vi "setup_id_from_ctlref.vi"(6 "error in":errorcluster, 7 "Ctl Refnum":refnum<vi>) -> (0 "error out":errorcluster, 1 "setup ID":u16)   [LabVIEW 2016]
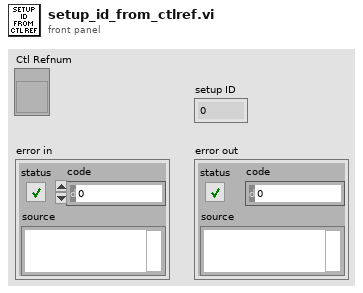
[diagram p1: front panel]
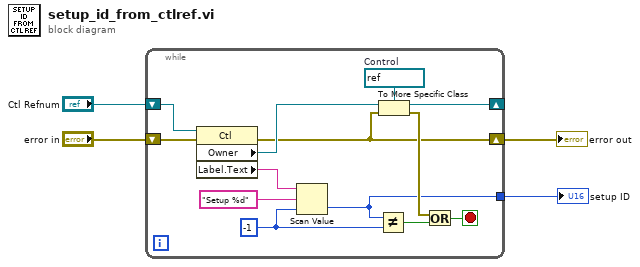
[diagram p0: block diagram]
diagram:
  n1 = while {
    shift-right: [w16] -> _
    shift-left: "Ctl Refnum" -> [w14]
    shift-right: [w8] -> w2
    shift-left: "error in" -> [w15]
    tunnel: [w5] -> w3
    stop <- w11 stop-if-true
    w6 = -1 ("default (0 dbl)")
    w17 = refnum<vi> refnum  # Control
    n2 = property class="Ctl"(reference=w14, error in=w15) -> (error out=w8:errorcluster, "Owner"=w10:refnum<vi>, "Label.Text"=w7:string)  [unwired: 1 out]
    n3 = Scan Value(string=w7, format string="Setup %d", default (0 dbl)=w6) -> (value=w5:i32)  [unwired: 1 out]
    n4 = Not Equal?(x=w5, y=w6) -> (x != y?=w13:bool)
    n5 = To More Specific Class(target class=w17, reference=w10, error in=w8) -> (specific class reference=w16:refnum<vi>, error out=w12:errorcluster)
    n6 = Or(x=w12, y=w13) -> (x .or. y?=w11:bool)
  }
  "setup ID" <- w3
  "error out" <- w2
